vi "Main.vi"() -> ()   [LabVIEW 2021, in "Example Plugin.lvlib"]
doc: "This template is for the Queued Message Handler design pattern.\n\nThe Event Handling Loop generates messages based on user interface actions.\n\nThe Message Handling Loop processes messages generated by the Event Handling Loop, or by other messages. The messages are string values, so new messages can be added easily to the Message Cases case structure in the Message Handling Loop. Each message cluster can also provide an optional value for Message Data, which is a variant that can be converted to whatever message-specific data is required."
uses:
  Example Plugin.lvlib
  <vilib>/Plug-In SDKs/InstrumentStudio SDK/InstrumentStudioPluginSDK.lvlibp/Plugin Events Enum.ctl
  controls/Configuration.ctl
  377644f2-3ba0-40c2-9637-345728516e3e.vi
  dd0e9e37-20d8-45cf-b11e-f419cd56f172.vi
  377644f2-3ba0-40c2-9637-345728516e3e.vi/6651a77e-856e-4bcd-af5a-c0c13b264cc1.vi
  dd0e9e37-20d8-45cf-b11e-f419cd56f172.vi/331b549c-fcf8-43d9-8a1e-5b3c0091a99c.vi
  subVIs/Message Queue/Enqueue Message (Single).vi
  <vilib>/JDP Science/JSONtext/JSON text to Variant.vi
  <vilib>/Utility/error.llb/Error Cluster From Error Code.vi
  <vilib>/JDP Science/JSONtext/Variant to JSON Text.vi
  <vilib>/JDP Science/JSONtext/LVClass Serializer/JSONtext LVClass Serializer.lvclass
  <vilib>/ErrorRing/Error Ring.xnode
  <vilib>/Plug-In SDKs/InstrumentStudio SDK/InstrumentStudioPluginSDK.lvlibp/Plugin Session.lvclass
  <vilib>/Plug-In SDKs/InstrumentStudio SDK/InstrumentStudioPluginSDK.lvlibp
panel:
  in  "Tab Control":T1(tab)
  out "Project Path":path
  in  "Run Write":string
  in  "Write Run Time Config":bool
  in  "Edit Write":string
  in  "Write Edit Time Config":bool
  out "Run Read":string
  in  "Read Run Time Config":bool
  out "Edit Read":string
  in  "Read Edit Time Config":bool
  in  "Read Project Path":bool
  in  "Running":bool
  out "Event Record":i32(listbox)
  in  "Session Id":u64
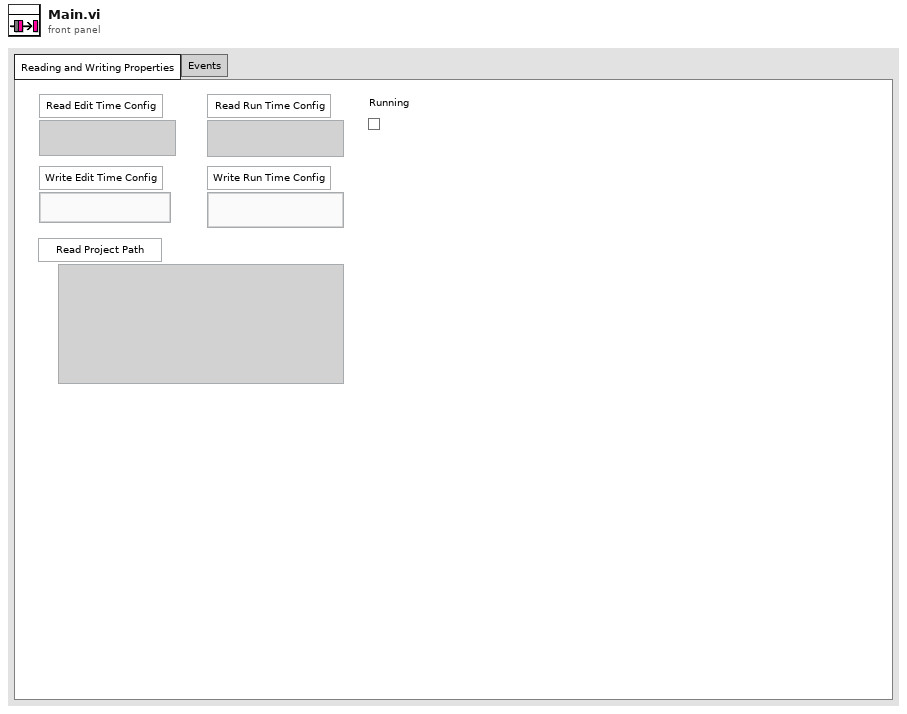
[diagram p1: front panel]
types:
  T1 = enum32{"Reading and Writing Properties", "Events"}
  T2 = typedef "Example Plugin.lvlib/Configuration.ctl" = cluster{"Edit Time Config":string, "Run Time Config":string, "Project Path":path}
  T3 = typedef "InstrumentStudioPluginSDK.lvlibp/Plugin Events Enum.ctl" = enum16{"Shutdown", "Project Saved", "Stop All Outputs"}
  T4 = typedef "InstrumentStudioPluginSDK.lvlibp/Event Registration Refnum.ctl" = refnum<event-registration>
  T5 = typedef "Example Plugin.lvlib/All Message Queues.ctl" = cluster{"UI":refnum<queue>}
  T6 = cluster{"Event Refnum":T4, "Event Registration Refnum":refnum<event-registration>}
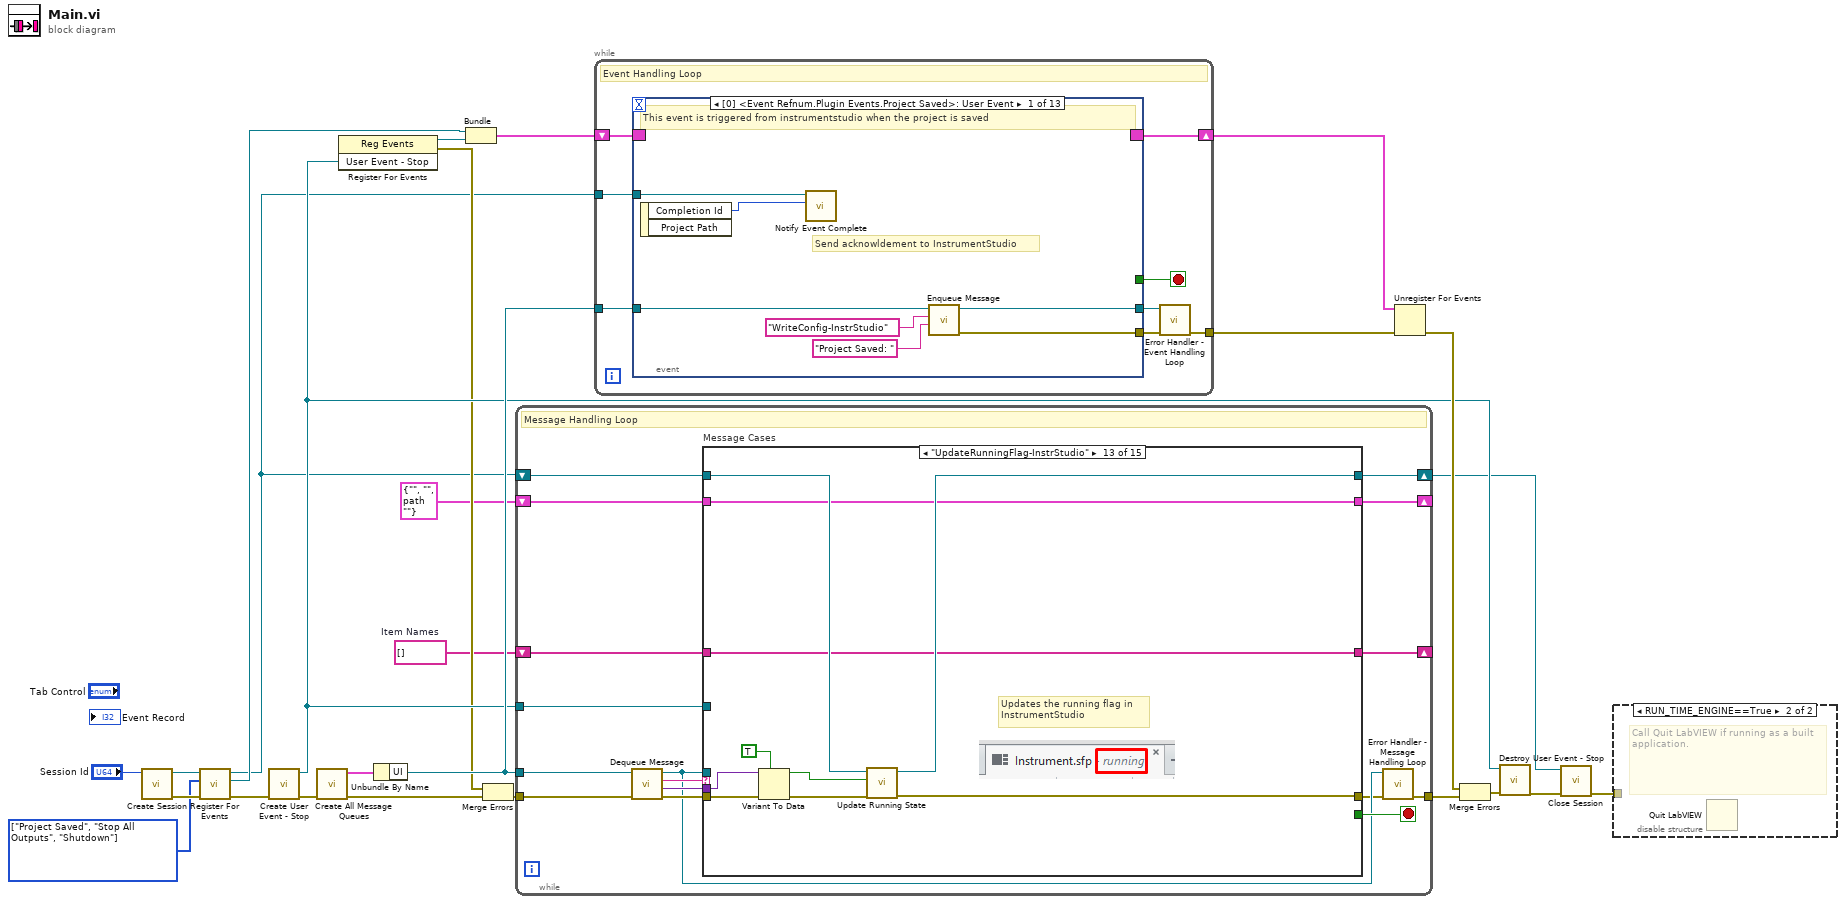
[diagram p0: block diagram]
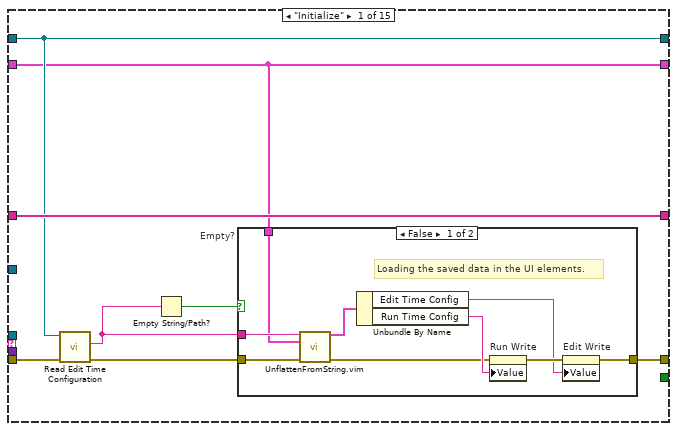
[diagram p3: hidden frame]
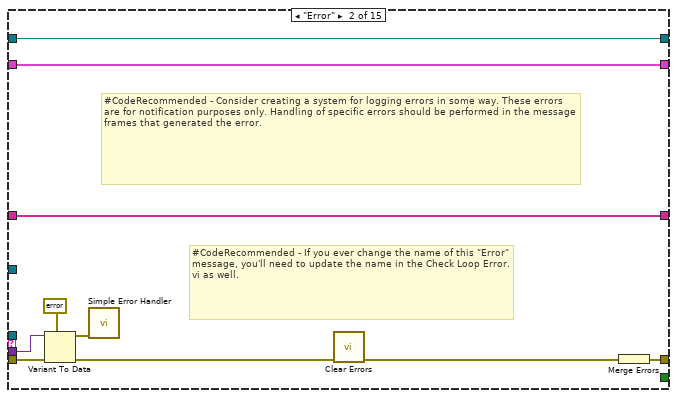
[diagram p5: hidden frame]
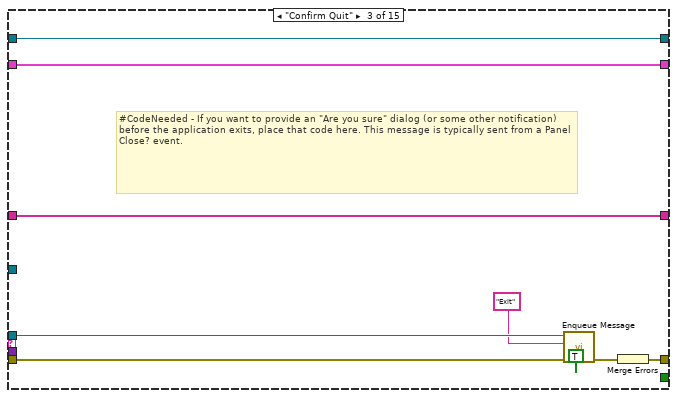
[diagram p6: hidden frame]
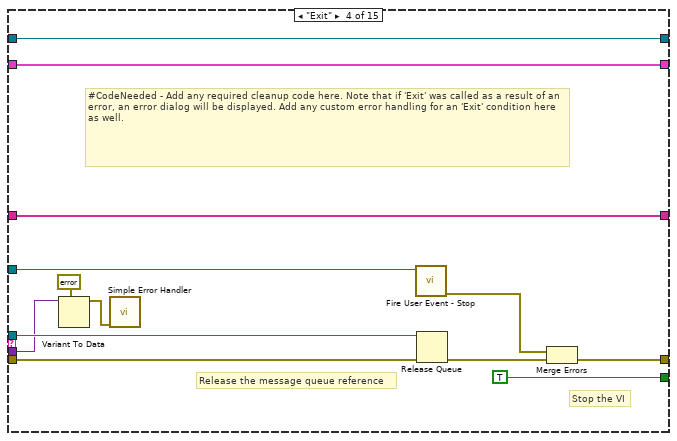
[diagram p7: hidden frame]
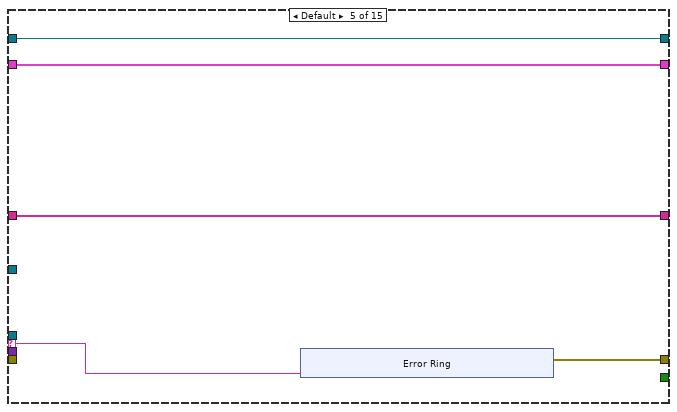
[diagram p8: hidden frame]
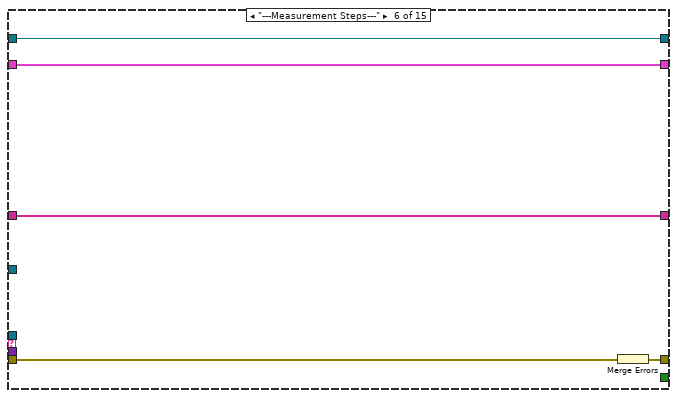
[diagram p9: hidden frame]
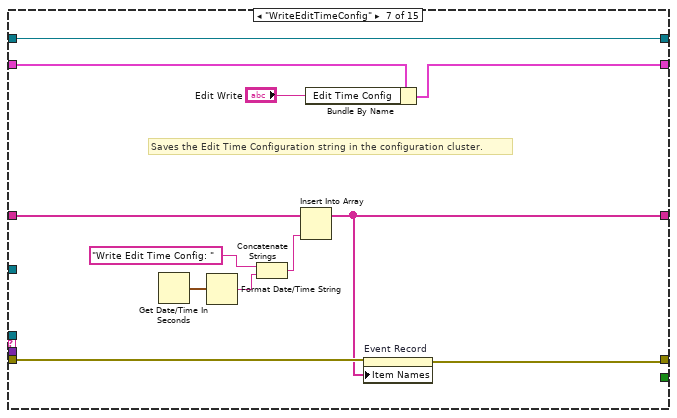
[diagram p10: hidden frame]
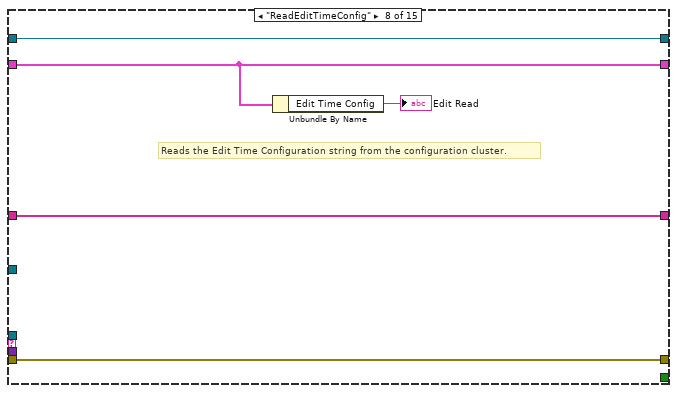
[diagram p11: hidden frame]
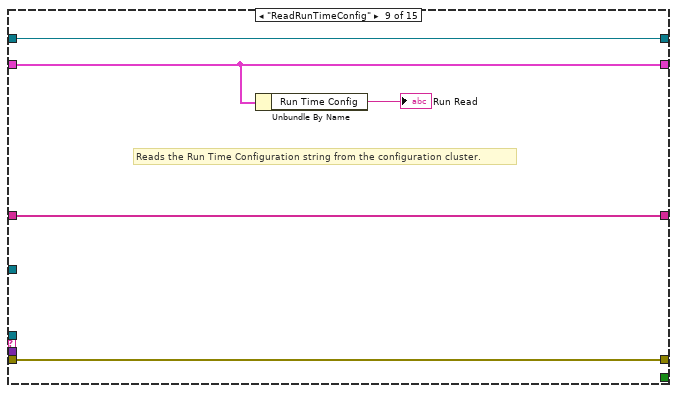
[diagram p12: hidden frame]
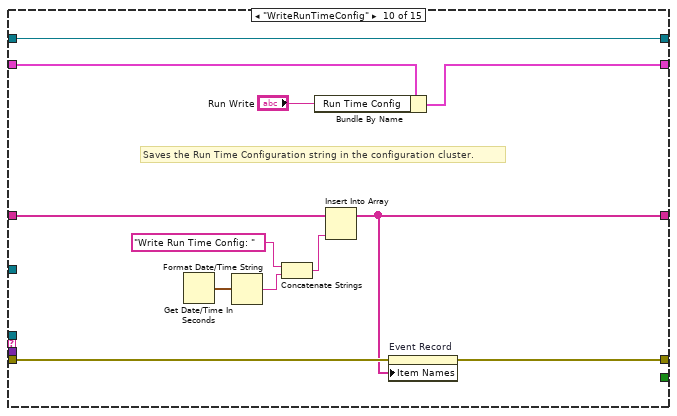
[diagram p13: hidden frame]
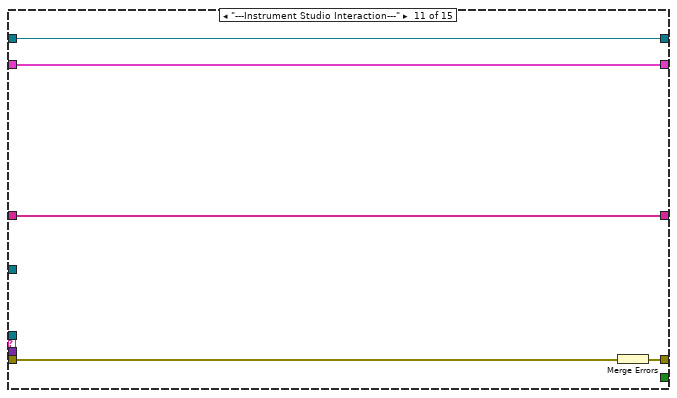
[diagram p14: hidden frame]
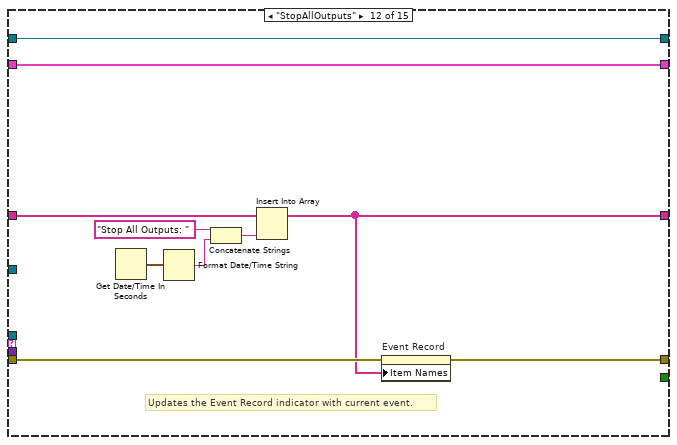
[diagram p15: hidden frame]
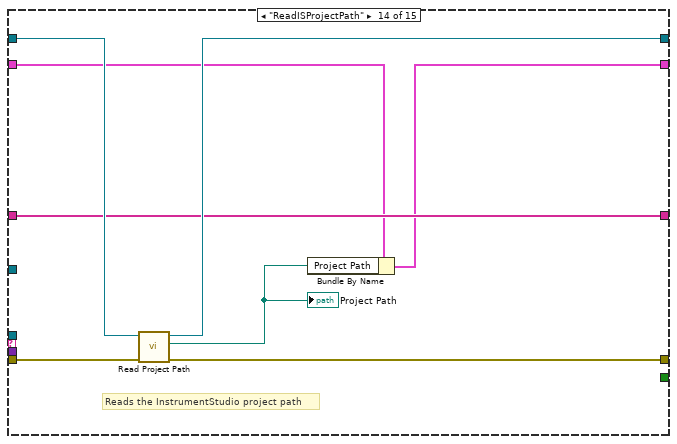
[diagram p16: hidden frame]
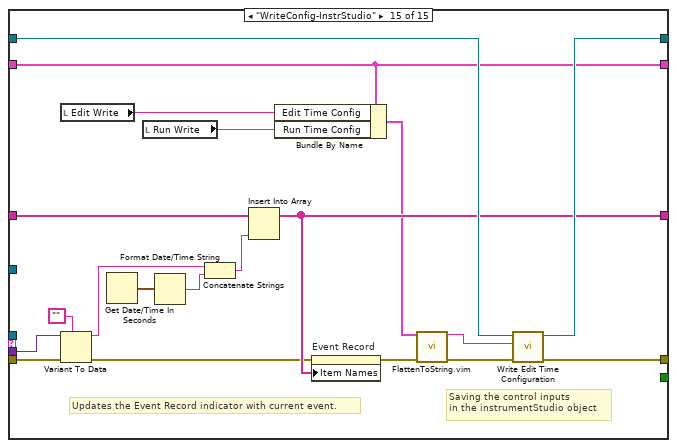
[diagram p17: hidden frame]
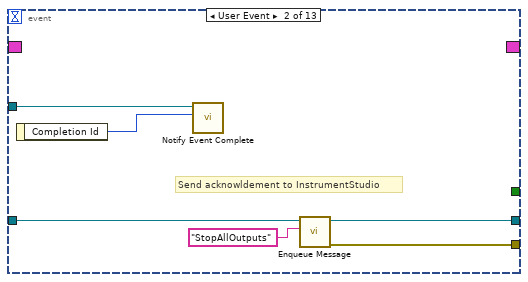
[diagram p18: hidden frame]
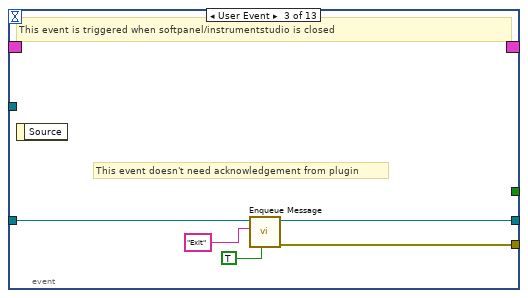
[diagram p19: hidden frame]
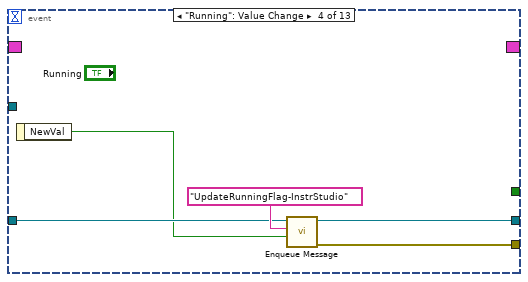
[diagram p20: hidden frame]
diagram:
  w1 = string[] []  # Item Names
  w10 = T3[] [enum."Project Saved", enum."Stop All Outputs", enum."Shutdown"] items=["Shutdown", "Project Saved", "Stop All Outputs"] ("Events To Register")
  n1 = call <vilib>:"Create Session.vi"("Session Id"="Session Id") -> ("error out"=w13:errorcluster, "Session out"=w11:refnum<class "Plugin Session.lvclass">)  [unwired: 6 in, 3 out]
  n2 = call <vilib>:"Register For Events.vi"("error in (no error)"=w13, "Events To Register"=w10, "Session in"=w11) -> ("error out"=w12:errorcluster, "Event Refnum"=w7:T4, "Session out"=w3:refnum<class "Plugin Session.lvclass">)  [unwired: 6 in]
  n3 = call "Create User Event - Stop.vi"("error in (no error)"=w12) -> ("error out"=w22:errorcluster, "User Event - Stop"=w17:refnum<user-event>)  [unwired: 9 in]
  n4 = call "Create All Message Queues.vi"("error in (no error)"=w22) -> ("error out"=w26:errorcluster, "Message Queues out"=w25:T5)  [unwired: 9 in]
  n5 = register-events(w17) -> (reference out=w9:refnum<event-registration>, error out=w15:errorcluster)  [unwired: 2 in]
  n6 = Unbundle By Name(w25) -> ("UI"=w23:refnum<queue>)
  n7 = Bundle("Event Refnum"=w7, "Event Registration Refnum"=w9) -> (w8:T6)  [unwired: 1 in]
  n8 = Merge Errors(w15, w26) -> (w16:errorcluster)
  n9 = while {
    tunnel: w23 -> [w36]
    tunnel: w17 -> [w41]
    tunnel: w16 -> [w40]
    tunnel: [w34] -> w24
    shift-right: [w31] -> w6
    shift-left: w3 -> [w32]
    shift-right: [w30] -> _
    shift-left: T2 {"Edit Time Config"="", "Run Time Config"="", "Project Path"=path ""} ("Configuration") -> [w29]
    shift-right: [w27] -> _
    shift-left: w1 -> [w28]
    stop <- w42 stop-if-true
    # "Message Handling Loop"
    n10 = call "Dequeue Message.vi"("error in (no error)"=w40, "Message Queue"=w36) -> ("error out"=w39:errorcluster, "Message Data"=w37:variant, "Message"=w38:string, "dup Message Queue"=w35:refnum<queue>)  [unwired: 6 in]
    n11 = case "Message Cases" shown="\"UpdateRunningFlag-InstrStudio\"" w38 {
      selector: w38 -> [_ _ _ _ w96 _ _ _ _ _ _ _ _ _ _]
      tunnel: w35 -> [_ _ w76 w92 _ _ _ _ _ _ _ _ _ _ _]
      tunnel: w39 -> [w46 w70 w79 w86 _ w109 w114 w126 w131 w136 w148 w150 w165 w175 w182]
      tunnel: [w50 w65 w78 w89 w97 w108 w113 w126 w131 w135 w147 w151 w166 w173 w194] -> w33
      tunnel: [_ _ _ TRUE _ _ _ _ _ _ _ _ _ _ _] -> w42
      tunnel: w37 -> [_ w69 _ w83 _ _ _ _ _ _ _ _ w164 _ w184]
      tunnel: w41 -> [_ _ _ w88 _ _ _ _ _ _ _ _ _ _ _]
      tunnel: w32 -> [w44 w64 w73 w82 w95 w107 w121 w125 w130 w143 w146 w158 w168 w176 w196]
      tunnel: [w44 w64 w73 w82 w95 w107 w121 w125 w130 w143 w146 w158 w167 w174 w195] -> w31
      tunnel: [w43 w63 w72 w81 w94 w106 w120 w123 w128 w142 w145 w157 w160 w170 w179] -> w30
      tunnel: w29 -> [w43 w63 w72 w81 w94 w106 w119 w123 w128 w141 w145 w157 w160 w169 w179]
      tunnel: w28 -> [w45 w61 w71 w80 w93 w105 w112 w124 w129 w134 w144 w152 w159 w172 w187]
      tunnel: [w45 w61 w71 w80 w93 w105 w111 w124 w129 w133 w144 w149 w159 w172 w186] -> w27
      frame "Initialize" {
        # "Initialize - All initialization work should take place in this message, since other loops can potentially enqueue messages that execute immediately after this one."
        n12 = call <vilib>:"Read Edit Time Configuration.vi"("error in (no error)"=w46, "Session in"=w44) -> ("error out"=w47:errorcluster, "Edit Time Configuration"=w48:string)  [unwired: 7 in, 1 out]
        n13 = Empty String/Path?(string/path=w48) -> (empty?=w49:bool)
        n14 = case "Empty?" shown="False" w49 {
          tunnel: w43 -> [w58 _]
          tunnel: [w53 w60] -> w50
          tunnel: w47 -> [w57 w60]
          tunnel: w48 -> [w59 _]
          frame False {
            # "Loading the saved data in the UI elements."
            n15 = call "UnflattenFromString.vim"("Flattened Data"=w59, "Data Type"=w58, "error in"=w57) -> ("Data Out"=w51:T2, "error out"=w55:errorcluster)  [unwired: 11 in]
            n16 = Unbundle By Name(w51) -> ("Edit Time Config"=w52:string, "Run Time Config"=w56:string)
            n17 = property on="Run Write" class="Str"(error in=w55, "Value"=w56) -> (error out=w54:errorcluster)  [unwired: 1 in, 1 out]
            n18 = property on="Edit Write" class="Str"(error in=w54, "Value"=w52) -> (error out=w53:errorcluster)  [unwired: 1 in, 1 out]
          }
          frame True {
          }
        }
      }
      frame "Error" {
        # "#CodeRecommended - If you ever change the name of this \"Error\" message, you'll need to update the name in the Check Loop Error.vi as well."
        # "#CodeRecommended - Consider creating a system for logging errors in some way. These errors are for notification purposes only. Handling of specific errors should be performed in the message frames that generated the error."
        # "Error - Display an error dialog. This message is sent by the \"Error Handler\" VIs at the end of other loops in this application."
        n19 = Variant To Data(error in=w70, type=errorcluster {"status"=FALSE, "code"=0, "source"=""} ("error constant"), Variant=w69) -> (data=w67:errorcluster, error out=w66:errorcluster)
        n20 = call <vilib>:"Simple Error Handler.vi"("error in (no error)"=w67) -> ()  [unwired: 4 in, 5 out]
        n21 = call <vilib>:"Clear Errors.vi"("error in (no error)"=w66) -> ("error out"=w62:errorcluster)  [unwired: 5 in, 1 out]
        n22 = Merge Errors(w62) -> (w65:errorcluster)
      }
      frame "Confirm Quit" {
        # "#CodeNeeded - If you want to provide an \"Are you sure\" dialog (or some other notification) before the application exits, place that code here. This message is typically sent from a Panel Close? event."
        # "Confirm Quit - Message that can confirm whether or not the user wants to exit the application."
        n23 = call-poly "Enqueue Message.vi"("Priority Message? (F)"=TRUE, "error in (no error)"=w79, "Message"="Exit", "Message Queue"=w76) -> ("error out"=w77:errorcluster)  [unwired: 6 in, 1 out]
        n24 = Merge Errors(w77) -> (w78:errorcluster)
      }
      frame "Exit" {
        # "Stop the VI"
        # "Release the message queue reference"
        # "#CodeNeeded - Add any required cleanup code here. Note that if 'Exit' was called as a result of an error, an error dialog will be displayed. Add any custom error handling for an 'Exit' condition here as well."
        # "Exit - Exit the application."
        n25 = Variant To Data(type=errorcluster {"status"=FALSE, "code"=0, "source"=""} ("error constant"), Variant=w83) -> (data=w84:errorcluster)  [unwired: 1 in, 1 out]
        n26 = call <vilib>:"Simple Error Handler.vi"("error in (no error)"=w84) -> ()  [unwired: 4 in, 5 out]
        n27 = call "Fire User Event - Stop.vi"("User Event - Stop"=w88) -> ("error out"=w87:errorcluster)  [unwired: 10 in]
        n28 = Release Queue(queue=w92, error in (no error)=w86) -> (error out=w90:errorcluster)  [unwired: 1 in, 2 out]
        n29 = Merge Errors(w87, w90) -> (w89:errorcluster)
      }
      frame Default {
        # "'Default' case only runs if there is a message that isn't defined in any of the other cases.  Output a programming error."
        n30 = xnode "Error Ring"("parameter 0"=w96) -> ("error out"=w97:errorcluster)
      }
      frame "---Measurement Steps---" {
        # "Duplicate this frame when creating new messages.  Change this comment in the duplicated frame to describe this message."
        n31 = Merge Errors(w109) -> (w108:errorcluster)
      }
      frame "WriteEditTimeConfig" {
        # "Saves the Edit Time Configuration string in the configuration cluster."
        n32 = Get Date/Time In Seconds() -> (seconds since 1Jan1904=w115:timestamp)
        n33 = Format Date/Time String(seconds (now)=w115) -> (date/time string=w117:string)  [unwired: 2 in]
        n34 = Concatenate Strings("Write Edit Time Config: " ("string"), w117) -> (w116:string)
        n35 = Insert Into Array(array=w112, new element=w116) -> (w111:string[])  [unwired: 1 in]
        n36 = Bundle By Name(cluster=w119, "Edit Time Config"="Edit Write") -> (w120:T2)
        n37 = property on="Event Record" class="LstBox (strict)"(error in=w114, "Item Names"=w111) -> (error out=w113:errorcluster)  [unwired: 1 in, 1 out]
      }
      frame "ReadEditTimeConfig" {
        # "Reads the Edit Time Configuration string from the configuration cluster."
        n38 = Unbundle By Name(w123) -> ("Edit Time Config"=→"Edit Read":string)
      }
      frame "ReadRunTimeConfig" {
        # "Reads the Run Time Configuration string from the configuration cluster."
        n39 = Unbundle By Name(w128) -> ("Run Time Config"=→"Run Read":string)
      }
      frame "WriteRunTimeConfig" {
        # "Saves the Run Time Configuration string in the configuration cluster."
        n40 = Get Date/Time In Seconds() -> (seconds since 1Jan1904=w137:timestamp)
        n41 = Format Date/Time String(seconds (now)=w137) -> (date/time string=w139:string)  [unwired: 2 in]
        n42 = Concatenate Strings("Write Run Time Config: " ("string"), w139) -> (w138:string)
        n43 = Bundle By Name(cluster=w141, "Run Time Config"="Run Write") -> (w142:T2)
        n44 = Insert Into Array(array=w134, new element=w138) -> (w133:string[])  [unwired: 1 in]
        n45 = property on="Event Record" class="LstBox (strict)"(error in=w136, "Item Names"=w133) -> (error out=w135:errorcluster)  [unwired: 1 in, 1 out]
      }
      frame "---Instrument Studio Interaction---" {
        # "Duplicate this frame when creating new messages.  Change this comment in the duplicated frame to describe this message."
        n46 = Merge Errors(w148) -> (w147:errorcluster)
      }
      frame "StopAllOutputs" {
        # "Updates the Event Record indicator with current event."
        n47 = Get Date/Time In Seconds() -> (seconds since 1Jan1904=w153:timestamp)
        n48 = Format Date/Time String(seconds (now)=w153) -> (date/time string=w155:string)  [unwired: 2 in]
        n49 = Concatenate Strings("Stop All Outputs: ", w155) -> (w154:string)
        n50 = Insert Into Array(array=w152, new element=w154) -> (w149:string[])  [unwired: 1 in]
        n51 = property on="Event Record" class="LstBox (strict)"(error in=w150, "Item Names"=w149) -> (error out=w151:errorcluster)  [unwired: 1 in, 1 out]
      }
      frame "UpdateRunningFlag-InstrStudio" {
        # "Updates the running flag in \nInstrumentStudio"
        n52 = Variant To Data(error in=w165, type=TRUE, Variant=w164) -> (data=w162:bool, error out=w161:errorcluster)
        n53 = call <vilib>:"Update Running State.vi"("error in (no error)"=w161, "Is Running"=w162, "Plugin Session in"=w168) -> ("error out"=w166:errorcluster, "Plugin Session out"=w167:refnum<class "Plugin Session.lvclass">)  [unwired: 7 in]
      }
      frame "ReadISProjectPath" {
        # "Reads the InstrumentStudio project path"
        n54 = call <vilib>:"Read Project Path.vi"("error in (no error)"=w175, "Session in"=w176) -> ("error out"=w173:errorcluster, "Project Path"=w171:path, "Session out"=w174:refnum<class "Plugin Session.lvclass">)  [unwired: 7 in]
        "Project Path" <- w171
        n55 = Bundle By Name(cluster=w169, "Project Path"=w171) -> (w170:T2)
      }
      frame "WriteConfig-InstrStudio" {
        # "Updates the Event Record indicator with current event."
        # "Saving the control inputs\nin the instrumentStudio object"
        n56 = local read "Edit Write"() -> (w178:string)
        n57 = Variant To Data(error in=w182, type="", Variant=w184) -> (data=w181:string, error out=w183:errorcluster)
        n58 = Get Date/Time In Seconds() -> (seconds since 1Jan1904=w189:timestamp)
        n59 = local read "Run Write"() -> (w177:string)
        n60 = Format Date/Time String(seconds (now)=w189) -> (date/time string=w191:string)  [unwired: 2 in]
        n61 = Concatenate Strings(w181, w191) -> (w190:string)
        n62 = Insert Into Array(array=w187, new element=w190) -> (w186:string[])  [unwired: 1 in]
        n63 = Bundle By Name(cluster=w179, "Edit Time Config"=w178, "Run Time Config"=w177) -> (w180:T2)
        n64 = property on="Event Record" class="LstBox (strict)"(error in=w183, "Item Names"=w186) -> (error out=w188:errorcluster)  [unwired: 1 in, 1 out]
        n65 = call "FlattenToString.vim"("Anything"=w180, "error in"=w188) -> ("Flattened Data"=w193:string, "error out"=w192:errorcluster)  [unwired: 12 in]
        n66 = call <vilib>:"Write Edit Time Configuration.vi"("error in (no error)"=w192, "Edit Time Configuration"=w193, "Session in"=w196) -> ("error out"=w194:errorcluster, "Session out"=w195:refnum<class "Plugin Session.lvclass">)  [unwired: 7 in]
      }
    }
    n67 = call "Error Handler - Message Handling Loop.vi"("error in (no error)"=w33, "Message Queue"=w35) -> ("dup error in"=w34:errorcluster)  [unwired: 8 in, 1 out]
  }
  n68 = while {
    tunnel: w23 -> [w204]
    shift-right: [w202] -> w19
    shift-left: w8 -> [w203]
    tunnel: [w198] -> w18
    tunnel: w3 -> [w197]
    stop <- w200 stop-if-true
    # "Event Handling Loop"
    n69 = event shown="[0] <Event Refnum.Plugin Events.Project Saved>: User Event" {
      selector: w203 -> [_ _ _ _ _ _ _ _ _ _ _ _ _]
      dyn-events: [_ _ _ _ _ _ _ _ _ _ _ _ _] -> w202
      timeout: _ -> [_ _ _ _ _ _ _ _ _ _ _ _ _]
      tunnel: [_ _ _ _ _ _ _ _ _ _ _ _ TRUE ("Discard?")] -> w200
      tunnel: w204 -> [w208 w215 w218 w226 w230 w234 w238 w240 w243 w245 w252 w254 w256]
      tunnel: [w206 w212 w219 w224 _ w233 _ _ _ _ w251 _ _] -> w201
      tunnel: [w207 w213 w220 w225 w231 w235 w237 w239 w242 w246 w250 w254 w256] -> w199
      tunnel: w197 -> [w211 w217 _ _ _ _ _ _ _ _ _ _ _]
      event User Event {
        # "Send acknowldement to InstrumentStudio"
        # "This event is triggered from instrumentstudio when the project is saved"
        n70 = event-data() -> ("Completion Id"=w210:i64)  [unwired: 1 in, 1 out]
        n71 = call <vilib>:"Notify Event Complete.vi"("Completion Id"=w210, "Session in"=w211) -> ()  [unwired: 8 in, 2 out]
        n72 = call-poly "Enqueue Message.vi"("Message Data"="Project Saved: " ("Message"), "Message"="WriteConfig-InstrStudio", "Message Queue"=w208) -> ("error out"=w206:errorcluster, "dup Message Queue"=w207:refnum<queue>)  [unwired: 7 in]
      }
      event User Event {
        # "Send acknowldement to InstrumentStudio"
        n73 = event-data() -> ("Completion Id"=w216:i64)  [unwired: 1 in]
        n74 = call <vilib>:"Notify Event Complete.vi"("Completion Id"=w216, "Session in"=w217) -> ()  [unwired: 8 in, 2 out]
        n75 = call-poly "Enqueue Message.vi"("Message"="StopAllOutputs", "Message Queue"=w215) -> ("error out"=w212:errorcluster, "dup Message Queue"=w213:refnum<queue>)  [unwired: 8 in]
      }
      event User Event {
        # "This event doesn't need acknowledgement from plugin"
        # "This event is triggered when softpanel/instrumentstudio is closed"
        n76 = event-data() -> ()  [unwired: 1 in, 1 out]
        n77 = call-poly "Enqueue Message.vi"("Priority Message? (F)"=TRUE, "Message"="Exit", "Message Queue"=w218) -> ("error out"=w219:errorcluster, "dup Message Queue"=w220:refnum<queue>)  [unwired: 7 in]
      }
      event "Running": Value Change {
        n78 = event-data() -> ("NewVal"=w223:bool)  [unwired: 1 in]
        n79 = call-poly "Enqueue Message.vi"("Message Data"=w223, "Message"="UpdateRunningFlag-InstrStudio", "Message Queue"=w226) -> ("error out"=w224:errorcluster, "dup Message Queue"=w225:refnum<queue>)  [unwired: 7 in]
      }
      event "Edit Write", "Run Write": Value Change {
        n80 = event-data() -> ()  [unwired: 1 in, 1 out]
        n81 = call-poly "Enqueue Message.vi"("Message Data"="Edit/Run Write: ", "Message"="WriteConfig-InstrStudio", "Message Queue"=w230) -> ("dup Message Queue"=w231:refnum<queue>)  [unwired: 7 in, 1 out]
      }
      event "Read Project Path": Value Change {
        n82 = event-data() -> ()  [unwired: 1 in, 1 out]
        n83 = call-poly "Enqueue Message.vi"("Message"="ReadISProjectPath", "Message Queue"=w234) -> ("error out"=w233:errorcluster, "dup Message Queue"=w235:refnum<queue>)  [unwired: 8 in]
      }
      event "Write Edit Time Config": Value Change {
        # "Enqueues WriteEditTimeConfig state to the queue driver."
        n84 = event-data() -> ()  [unwired: 1 in, 1 out]
        n85 = call-poly "Enqueue Message.vi"("Message"="WriteEditTimeConfig", "Message Queue"=w238) -> ("dup Message Queue"=w237:refnum<queue>)  [unwired: 8 in, 1 out]
      }
      event "Read Edit Time Config": Value Change {
        # "Enqueues ReadEditTimeConfig state to the queue driver."
        n86 = event-data() -> ()  [unwired: 1 in, 1 out]
        n87 = call-poly "Enqueue Message.vi"("Message"="ReadEditTimeConfig", "Message Queue"=w240) -> ("dup Message Queue"=w239:refnum<queue>)  [unwired: 8 in, 1 out]
      }
      event "Read Run Time Config": Value Change {
        # "Enqueues ReadRunTimeConfig state to the queue driver."
        n88 = event-data() -> ()  [unwired: 1 in, 1 out]
        n89 = call-poly "Enqueue Message.vi"("Message"="ReadRunTimeConfig", "Message Queue"=w243) -> ("dup Message Queue"=w242:refnum<queue>)  [unwired: 8 in, 1 out]
      }
      event "Write Run Time Config": Value Change {
        # "Enqueues WriteRunTimeConfig state to the queue driver."
        n90 = event-data() -> ()  [unwired: 1 in, 1 out]
        n91 = call-poly "Enqueue Message.vi"("Message"="WriteRunTimeConfig", "Message Queue"=w245) -> ("dup Message Queue"=w246:refnum<queue>)  [unwired: 8 in, 1 out]
      }
      event Panel Close? {
        # "Send the 'Confirm Quit' message if the user closes the panel of the VI. Discard the event so the 'Confirm Quit' message has a chance to run."
        n92 = event-data() -> ()  [unwired: 1 in, 1 out]
        n93 = call-poly "Enqueue Message.vi"("Priority Message? (F)"=TRUE, "Message"="Confirm Quit", "Message Queue"=w252) -> ("error out"=w251:errorcluster, "dup Message Queue"=w250:refnum<queue>)  [unwired: 7 in]
        n94 = event-data("Discard?"=TRUE) -> ()  [unwired: 1 in, 1 out]
      }
      event Application Instance Close {
        # "#CodeRecommended - When a project closes, all VIs within that project are aborted and leave memory. However, any code placed in this event frame is guaranteed to run to completion, so add any cleanup code that absolutely must happen here."
        n95 = event-data() -> ()  [unwired: 1 in, 1 out]
      }
      event User Event {
        # "The Message Handling Loop processed an \"Exit\" message, which fired this event to stop the Event Handling Loop."
        n96 = event-data() -> ()  [unwired: 1 in, 1 out]
      }
    }
    n97 = call "Error Handler - Event Handling Loop.vi"("error in (no error)"=w201, "Message Queue"=w199) -> ("dup error in"=w198:errorcluster)  [unwired: 8 in, 1 out]
  }
  n98 = Unregister For Events(event registration refnum=w19, error in=w18) -> (error out=w20:errorcluster)
  n99 = Merge Errors(w20, w24) -> (w21:errorcluster)
  n100 = call "Destroy User Event - Stop.vi"("error in (no error)"=w21, "User Event - Stop"=w17) -> ("error out"=w5:errorcluster)  [unwired: 9 in]
  n101 = call <vilib>:"Close Session.vi"("error in (no error)"=w5, "Session in"=w6) -> ("error out"=w4:errorcluster)  [unwired: 9 in]
  n102 = disable-structure shown="RUN_TIME_ENGINE==True" {
    disable-tunnel: w4 -> [_ _]
    frame condition #0 (active) {
    }
    frame condition #1 {
      # "Call Quit LabVIEW if running as a built application."
      n103 = Quit LabVIEW() -> ()  [unwired: 1 in]
    }
  }
